vi "Rotation stage shgv8.vi"() -> ()   [LabVIEW 2020]
uses:
  <vilib>/Utility/error.llb/DialogType.ctl
  <vilib>/DAQmx/read.llb/DAQmx Read (Analog 1D Wfm NChan 1Samp).vi
  <vilib>/DAQmx/read.llb/DAQmx Read (Counter U32 1Chan 1Samp).vi
  <vilib>/DAQmx/create/channels.llb/DAQmx Create Channel (CI-Count Edges).vi
  <vilib>/DAQmx/miscellaneous.llb/DAQmx Fill In Error Info.vi
  <vilib>/DAQmx/create/channels.llb/DAQmx Create Channel (AI-Current-Basic).vi
  <vilib>/DAQmx/configure/timing.llb/DAQmx Timing (Sample Clock).vi
  <resource>/objmgr/daqmx.rc
panel:
  out "Actual Sample Rate":dbl=1000.0 format="%0.2f"
  out "data 2":waveform(dbl)[](graph)
  out "Consumer Iteration 3":i32=1109257
  in  "stop 4":bool
  out "Producer Iteration 3":i32=1109256
  out "error out 3":errorcluster
  out "Loop Time (ms) 3":u32=10
  in  "Stop":bool
  in  "Loop Time (ms)":u32=10
  out "Count":u32
  in  "Active Edge":i32(ring)=10171 items=["Rising"=10280, "Falling"=10171]
  in  "Input Terminal":tag="PFI8"
  in  "Counter":tag="Dev1/ctr0"
  in  "Trigger Type":T1(tab)
  in  "Edge":i32(ring)=10280 items=["Rising"=10280, "Falling"=10171]
  in  "Digital Trigger Source":tag
  in  "Pause When":i32(ring)=10192 items=["High"=10192, "Low"=10214]
  in  "Pause Trigger Source":tag
  in  "Count Reset Terminal":tag
  in  "Edge 2":i32(ring)=10280 items=["Rising"=10280, "Falling"=10171]
  in  "Rotation Angle (Degrees)":dbl=100.0 min=0.0
  in  "MG17Motor":refnum<k7>(container)
  # "To configure and use a trigger or the count reset you must have the necessary tab selected above.  Not all hardware supports the above options--refer to your device documentation for more info."
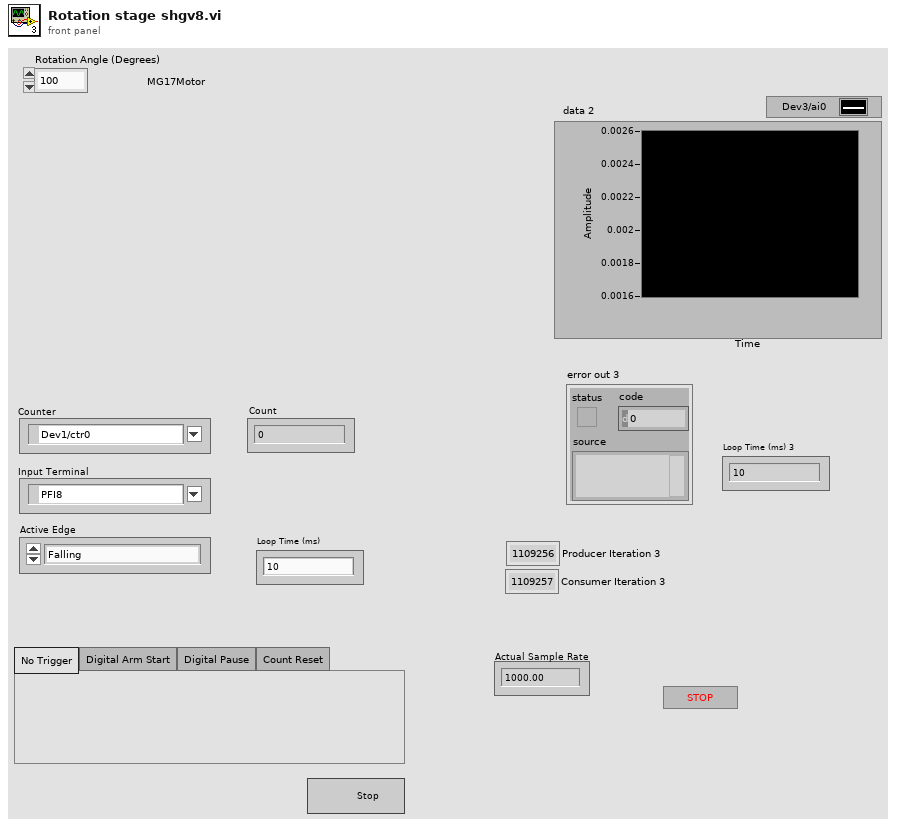
[diagram p1: front panel]
types:
  T1 = enum32{"No Trigger", "Digital Arm Start", "Digital Pause", "Count Reset"}
  T2 = enum16{"open", "open or create", "create or replace", "create", "open (read-only)"}
  T3 = typedef "DialogType.ctl" = u16
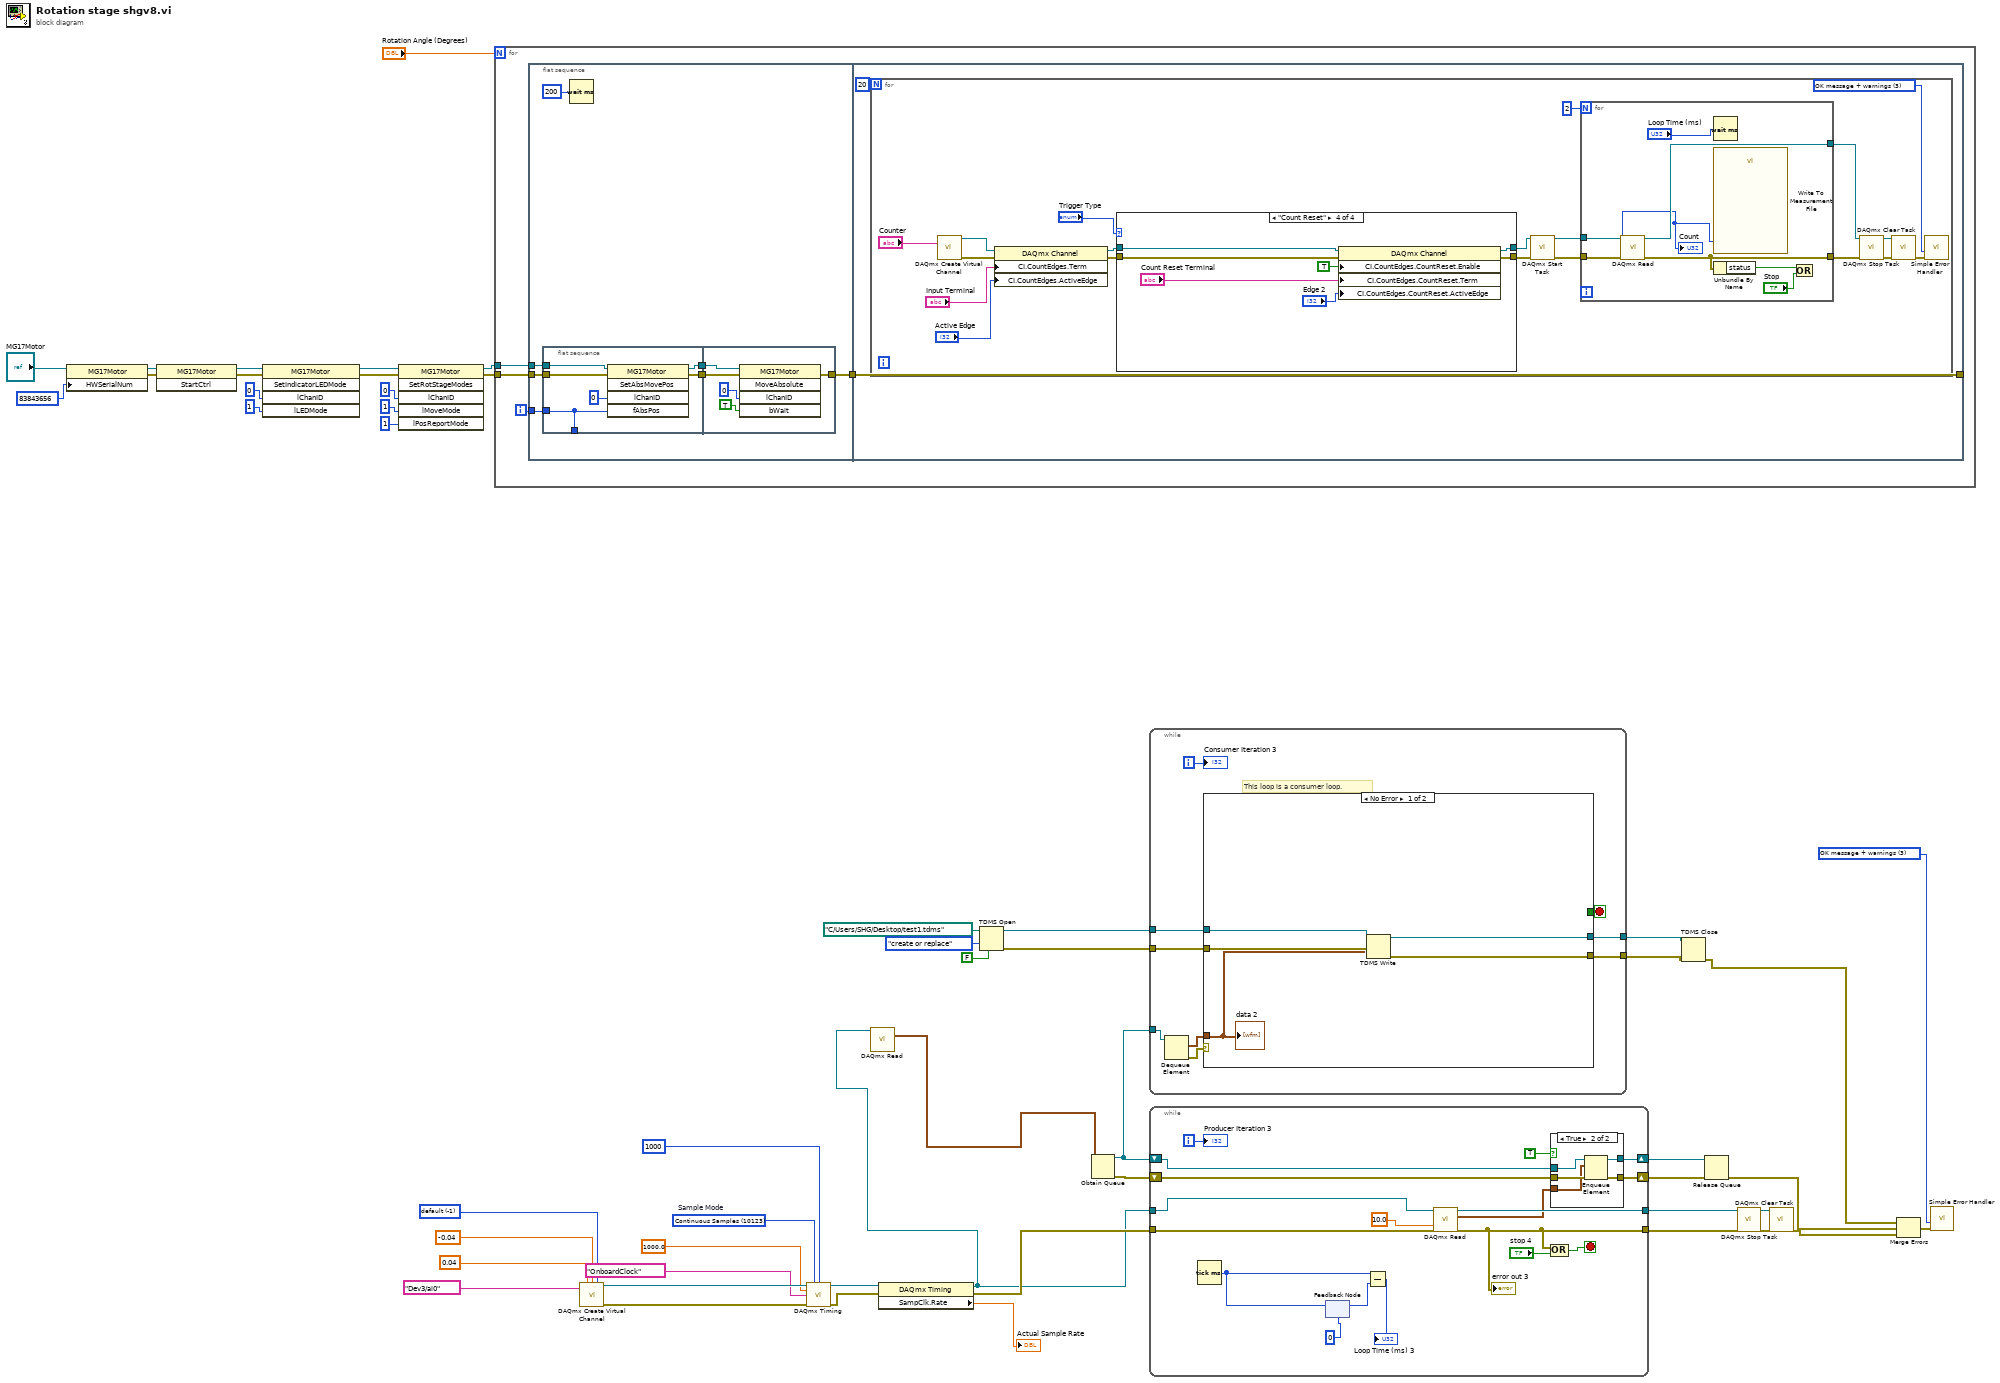
[diagram p0: block diagram]
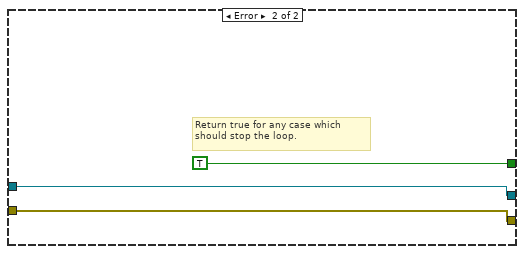
[diagram p2: hidden frame]
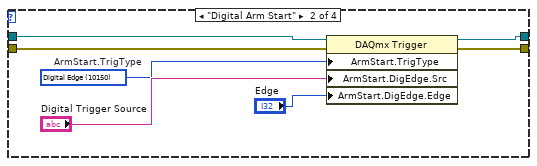
[diagram p5: hidden frame]
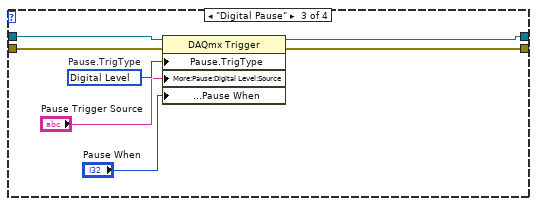
[diagram p6: hidden frame]
diagram:
  w6 = -1 items=["default"=-1, "RSE"=10083, "NRSE"=10078, "Differential"=10106, "Pseudodifferential"=12529] ("Terminal Configuration")
  w14 = 10123 items=["Finite Samples"=10178, "Continuous Samples"=10123, "Hardware Timed Single Point"=12522]  # Sample Mode
  w24 = T3 3 items=["no dialog", "OK message", "continue or stop message", "OK message + warnings", "continue/stop + warnings"] ("type of dialog (OK msg:1)")
  n1 = property class="MG17Motor"(reference="MG17Motor", "HWSerialNum"=83843656) -> (reference out=w51:refnum<k7>, error out=w50:errorcluster)  [unwired: 1 in]
  n2 = invoke class="MG17Motor" method="StartCtrl"(reference=w51, error in=w50) -> (reference out=w43:refnum<k7>, error out=w41:errorcluster)  [unwired: 1 in, 1 out]
  n3 = invoke class="MG17Motor" method="SetIndicatorLEDMode"(reference=w43, error in=w41, "lChanID"=0, "lLEDMode"=1) -> (reference out=w42:refnum<k7>, error out=w40:errorcluster)  [unwired: 1 in, 3 out]
  n4 = invoke class="MG17Motor" method="SetRotStageModes"(reference=w42, error in=w40, "lChanID"=0, "lMoveMode"=1, "lPosReportMode"=1) -> (reference out=w46:refnum<k7>, error out=w37:errorcluster)  [unwired: 1 in, 4 out]
  n5 = for {
    N: "Rotation Angle (Degrees)" -> [_]
    tunnel: w46 -> [w56]
    tunnel: w37 -> [w53]
    i -> [w54]
    n6 = flat-sequence {
      tunnel: w56 -> [w61]
      tunnel: w53 -> [w59]
      tunnel: [w58] -> w55
      tunnel: w54 -> [w60]
      tunnel: [w76] -> _
      tunnel: w55 -> [w76]
      frame #0 {
        n7 = flat-sequence {
          tunnel: [w64] -> _
          tunnel: w59 -> [w68]
          tunnel: w61 -> [w67]
          tunnel: [w66] -> w63
          tunnel: [w65] -> w62
          tunnel: w60 -> [w64]
          tunnel: w63 -> [w72]
          tunnel: w62 -> [w71]
          tunnel: [w70] -> w58
          frame #0 {
            n8 = invoke class="MG17Motor" method="SetAbsMovePos"(reference=w67, error in=w68, "lChanID"=0, "fAbsPos"=w64) -> (reference out=w65:refnum<k7>, error out=w66:errorcluster)  [unwired: 1 in, 3 out]
          }
          frame #1 {
            n9 = invoke class="MG17Motor" method="MoveAbsolute"(reference=w71, error in=w72, "lChanID"=0, "bWait"=TRUE) -> (error out=w70:errorcluster)  [unwired: 1 in, 4 out]
          }
        }
        n10 = Wait (ms)(milliseconds to wait=u32 200) -> ()  [unwired: 1 out]
      }
      frame #1 {
        n11 = for {
          N: 20 -> [_]
          w78 = T3 3 items=["no dialog", "OK message", "continue or stop message", "OK message + warnings", "continue/stop + warnings"] ("type of dialog (OK msg:1)")
          n12 = call-poly <vilib>:"DAQmx Create Virtual Channel.vi"("counter"="Counter") -> ("task out"=w86:refnum<k21>, "error out"=w85:errorcluster)  [unwired: 13 in]
          n13 = property class="DAQmx Channel"(reference=w86, error in=w85, "CI.CountEdges.Term"="Input Terminal", "CI.CountEdges.ActiveEdge"="Active Edge") -> (reference out=w83:refnum<k21>, error out=w84:errorcluster)
          n14 = case shown="\"Count Reset\"" "Trigger Type" {
            tunnel: w83 -> [w105 w112 w119 w126]
            tunnel: w84 -> [w104 w109 w116 w123]
            tunnel: [w105 w111 w118 w125] -> w93
            tunnel: [w104 w110 w117 w124] -> w92
            frame "No Trigger", Default {
            }
            frame "Digital Arm Start" {
              w106 = 10150 items=["Digital Edge"=10150, "None"=10230]  # ArmStart.TrigType
              n15 = property class="DAQmx Trigger"(reference=w112, error in=w109, "ArmStart.TrigType"=w106, "ArmStart.DigEdge.Src"="Digital Trigger Source", "ArmStart.DigEdge.Edge"="Edge") -> (reference out=w111:refnum<k21>, error out=w110:errorcluster)
            }
            frame "Digital Pause" {
              w115 = 10152 items=["Analog Level"=10101, "Analog Window"=10103, "Digital Level"=10152, "Digital Pattern"=10398, "None"=10230]  # Pause.TrigType
              n16 = property class="DAQmx Trigger"(reference=w119, error in=w116, "Pause.TrigType"=w115, "More:Pause:Digital Level:Source"="Pause Trigger Source", "More:Pause:Digital Level:Pause When"="Pause When") -> (reference out=w118:refnum<k21>, error out=w117:errorcluster)
            }
            frame "Count Reset" {
              n17 = property class="DAQmx Channel"(reference=w126, error in=w123, "CI.CountEdges.CountReset.Enable"=TRUE, "CI.CountEdges.CountReset.Term"="Count Reset Terminal", "CI.CountEdges.CountReset.ActiveEdge"="Edge 2") -> (reference out=w125:refnum<k21>, error out=w124:errorcluster)
            }
          }
          n18 = call <vilib>:"DAQmx Start Task.vi"("task/channels in"=w93, "error in"=w92) -> ("task out"=w91:refnum<k21>, "error out"=w90:errorcluster)  [unwired: 12 in]
          n19 = for {
            N: 2 -> [_]
            tunnel: w91 -> [w103]
            tunnel: w90 -> [w102]
            tunnel: [w100] -> w81
            tunnel: [w101] -> w82
            n20 = call-poly <vilib>:"DAQmx Read.vi"("task/channels in"=w103, "error in"=w102) -> ("task out"=w101:refnum<k21>, "data"=w96:u32, "error out"=w100:errorcluster)  [unwired: 11 in]
            "Count" <- w96
            n21 = Wait (ms)(milliseconds to wait="Loop Time (ms)") -> ()  [unwired: 1 out]
            n22 = call "Write To Measurement File"("Signals"=w96) -> ()  [unwired: 16 in, 3 out]
            n23 = Unbundle By Name(w100) -> ("status"=w99:bool)
            n24 = Or(x=w99, y="Stop") -> ()  [unwired: 1 out]
          }
          n25 = call <vilib>:"DAQmx Stop Task.vi"("task/channels in"=w82, "error in"=w81) -> ("task out"=w79:refnum<k21>, "error out"=w80:errorcluster)  [unwired: 12 in]
          n26 = call <vilib>:"DAQmx Clear Task.vi"("task in"=w79, "error in"=w80) -> ("error out"=w89:errorcluster)  [unwired: 13 in]
          n27 = call <vilib>:"Simple Error Handler.vi"("type of dialog (OK msg:1)"=w78, "error in (no error)"=w89) -> ()  [unwired: 3 in, 5 out]
        }
      }
    }
  }
  n28 = call-poly <vilib>:"DAQmx Create Virtual Channel.vi"("maximum value"=0.04 ("Max Voltage"), "minimum value"=-0.04 ("Min Voltage"), "input terminal configuration"=w6, "physical channels"=tag "Dev3/ai0" ("Physical Channel")) -> ("task out"=w12:refnum<k21>, "error out"=w13:errorcluster)  [unwired: 10 in]
  n29 = call-poly <vilib>:"DAQmx Timing.vi"("task/channels in"=w12, "sample mode"=w14, "samples per channel"=1000 ("Number of Samples"), "rate"=1000.0 ("Sample Rate"), "source"=tag "OnboardClock" ("Sample Clock Source"), "error in"=w13) -> ("task out"=w16:refnum<k21>, "error out"=w15:errorcluster)  [unwired: 8 in]
  n30 = property class="DAQmx Timing"(reference=w16, error in=w15) -> (reference out=w1:refnum<k21>, error out=w10:errorcluster, "SampClk.Rate"=→"Actual Sample Rate":dbl)
  n31 = call-poly <vilib>:"DAQmx Read.vi"("task/channels in"=w1) -> ("data"=w2:waveform(dbl)[])  [unwired: 12 in, 2 out]
  n32 = TDMS Open(6:FALSE ("disable buffering? (T)"), 10:T2."create or replace" ("operation (0:open)"), 11:path "C:/Users/SHG/Desktop/test1.tdms" ("file path")) -> (0:w26:errorcluster, 3:w28:refnum<k34>)  [unwired: 4 in]
  n33 = Obtain Queue(element data type=w2) -> (queue out=w36:refnum<queue>, error out=w35:errorcluster)  [unwired: 4 in, 1 out]
  n34 = while {
    tunnel: w36 -> [w135]
    tunnel: w28 -> [w130]
    tunnel: [w129] -> w27
    tunnel: w26 -> [w128]
    tunnel: [w127] -> w25
    i -> [w131]
    stop <- w132 stop-if-true
    # "This loop is a consumer loop."
    n35 = Dequeue Element(queue=w135) -> (element=w133:waveform(dbl)[], error out=w134:errorcluster)  [unwired: 2 in, 2 out]
    n36 = case shown="No Error" w134 {
      tunnel: w133 -> [w136 _]
      tunnel: [_ TRUE] -> w132
      tunnel: w130 -> [w140 w142]
      tunnel: [w139 w142] -> w129
      tunnel: w128 -> [w138 w141]
      tunnel: [w137 w141] -> w127
      frame No Error {
        n37 = TDMS Write(0:w140, 9:w136, 11:w138) -> (4:w139:refnum<k34>, 15:w137:errorcluster)  [unwired: 3 in, 2 out]
        "data 2" <- w136
      }
      frame Error {
        # "Return true for any case which should stop the loop."
      }
    }
    "Consumer Iteration 3" <- w131
  }
  n38 = while {
    shift-right: [w151] -> w33
    shift-left: w35 -> [w159]
    shift-right: [w160] -> w34
    shift-left: w36 -> [w161]
    tunnel: [w157] -> w30
    tunnel: [w150] -> w29
    tunnel: w10 -> [w156]
    tunnel: w1 -> [w155]
    i -> [w152]
    stop <- w148 stop-if-true
    n39 = Tick Count (ms)() -> (millisecond timer value=w147:u32)
    n40 = feedback #1(u32 0 ("millisecond timer value")) -> (w146:u32)
    n41 = feedback-in #1(w147) -> ()
    n42 = Subtract(x=w147, y=w146) -> (x-y=→"Loop Time (ms) 3":u32)
    n43 = call-poly <vilib>:"DAQmx Read.vi"("task/channels in"=w155, "timeout"=10.0, "error in"=w156) -> ("task out"=w157:refnum<k21>, "data"=w154:waveform(dbl)[], "error out"=w150:errorcluster)  [unwired: 10 in]
    "error out 3" <- w150
    n44 = case shown="True" TRUE ("Case Constant\n(See Context Help)") {
      tunnel: w161 -> [w163 w168]
      tunnel: [w163 w167] -> w160
      tunnel: w159 -> [w162 w166]
      tunnel: [w162 w165] -> w151
      tunnel: w154 -> [_ w164]
      frame False {
      }
      frame True {
        n45 = Enqueue Element(queue=w168, element=w164, error in (no error)=w166) -> (queue out=w167:refnum<queue>, error out=w165:errorcluster)  [unwired: 1 in, 1 out]
      }
    }
    n46 = Compound Arithmetic op=OR(w150, "stop 4") -> (w148:bool)
    "Producer Iteration 3" <- w152
  }
  n47 = TDMS Close(8:w25, 11:w27) -> (0:w20:errorcluster)  [unwired: 1 out]
  n48 = Release Queue(queue=w34, error in (no error)=w33) -> (error out=w19:errorcluster)  [unwired: 1 in, 2 out]
  n49 = call <vilib>:"DAQmx Stop Task.vi"("task/channels in"=w30, "error in"=w29) -> ("task out"=w31:refnum<k21>, "error out"=w32:errorcluster)  [unwired: 12 in]
  n50 = call <vilib>:"DAQmx Clear Task.vi"("task in"=w31, "error in"=w32) -> ("error out"=w18:errorcluster)  [unwired: 13 in]
  n51 = Merge Errors(w20, w19, w18) -> (w23:errorcluster)
  n52 = call <vilib>:"Simple Error Handler.vi"("type of dialog (OK msg:1)"=w24, "error in (no error)"=w23) -> ()  [unwired: 3 in, 5 out]
